vi "Check Valid UI Selection.vi"(8 "error in (no error)":errorcluster, 11 "Operator UI in":refnum<class "Measurement UI.lvclass">) -> (0 "error out":errorcluster, 3 "Operator UI out":refnum<class "Measurement UI.lvclass">)   [LabVIEW 2015, in "Measurement UI.lvlib" / "Measurement UI.lvclass"]
uses:
  Measurement UI.lvclass
  Measurement UI.lvclass/Measurement UI.ctl
  Accessors/Read Run.vi
  Accessors/Read Digitizer.vi
  Accessors/Read Function Generator.vi
  Accessors/Read Power Supply.vi
  Read Multimeter.vi
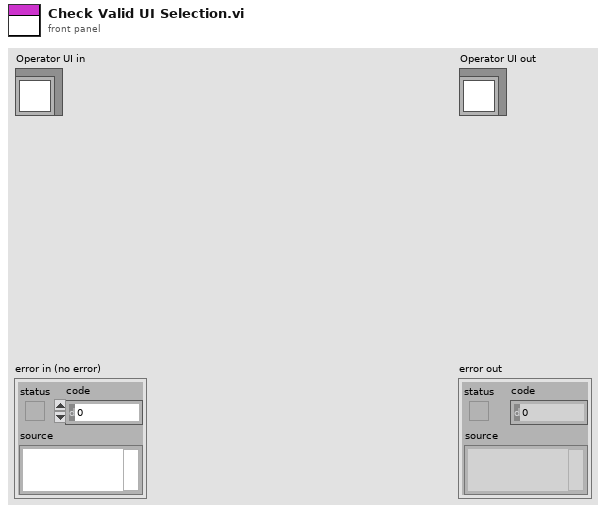
[diagram p1: front panel]
types:
  T1 = enum8{"Enabled", "Disabled", "Disabled and Grayed Out"}
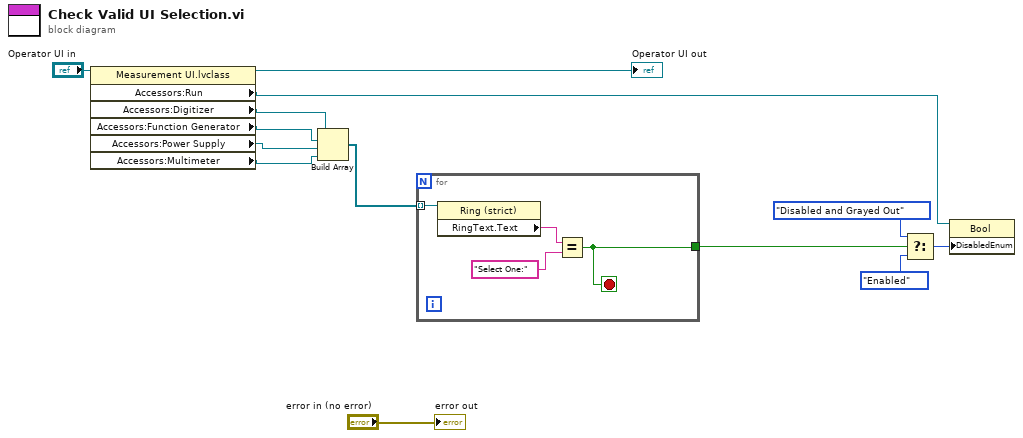
[diagram p0: block diagram]
diagram:
  n1 = property class="Measurement UI.lvclass"(reference="Operator UI in") -> (reference out=→"Operator UI out":refnum<class "Measurement UI.lvclass">, "Accessors:Run"=w1:refnum<vi>, "Accessors:Digitizer"=w2:refnum<vi>, "Accessors:Function Generator"=w3:refnum<vi>, "Accessors:Power Supply"=w4:refnum<vi>, "Accessors:Multimeter"=w5:refnum<vi>)  [unwired: 1 in, 1 out]
  n2 = Build Array(w2, w3, w4, w5) -> (w11:refnum<vi>[])
  n3 = for {
    tunnel: w11 -> [w17] mode=indexing
    tunnel: [w14] -> w9
    stop <- w14 stop-if-true
    n4 = property class="Ring (strict)"(reference=w17) -> ("RingText.Text"=w16:string)  [unwired: 1 in, 2 out]
    n5 = Equal?(x=w16, y="Select One:") -> (x = y?=w14:bool)
  }
  n6 = Select(t=T1."Disabled and Grayed Out" ("Disabled"), s=w9, f=T1."Enabled" ("Disabled")) -> (s? t:f=w10:T1)
  n7 = property class="Bool"(reference=w1, "DisabledEnum"=w10) -> ()  [unwired: 1 in, 2 out]
  "error out" <- "error in (no error)"
